vi "loadLVModule.vi"(0 "LV Module":refnum<k7>, 5 "VIPath":string, 11 "error in":errorcluster) -> (4 "LV Module(out)":refnum<k7>, 15 "error out":errorcluster)   [LabVIEW 2010]
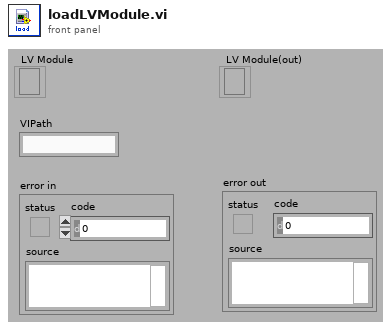
[diagram p1: front panel]
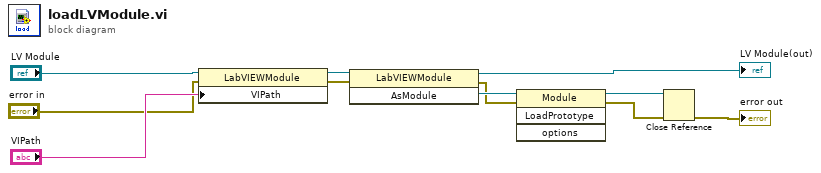
[diagram p0: block diagram]
diagram:
  n1 = property class="LabVIEWModule"(reference="LV Module", error in="error in", "VIPath"="VIPath") -> (reference out=w7:refnum<k7>, error out=w8:errorcluster)
  n2 = invoke class="LabVIEWModule" method="AsModule"(reference=w7, error in=w8) -> (reference out=→"LV Module(out)":refnum<k7>, error out=w3:errorcluster, "AsModule"=w4:refnum<k7>)  [unwired: 1 in]
  n3 = invoke class="Module" method="LoadPrototype"(reference=w4, error in=w3) -> (reference out=w2:refnum<k7>, error out=w1:errorcluster)  [unwired: 2 in, 2 out]
  n4 = Close Reference(reference=w2, error in (no error)=w1) -> (error out=→"error out":errorcluster)
